vi "SWERVE_TRAJECTORY_BEGIN.vi"(10 "gyroAngle":T2={"VALUE"=0.0, "COS"=1.0, "SIN"=0.0} {"SIN" format="%13.4f"; "COS" format="%13.4f"; "VALUE" format="%13.4f"}, 11 "Module Positions":T1[](array[typedef]) {"Angle"."SIN" format="%13.4f"; "Angle"."COS" format="%13.4f"; "Angle"."VALUE" format="%13.4f"}) -> ()   [LabVIEW 2019]
uses:
  <vilib>/Rock Robotics/WPI/ThirdParty/JAS_Junk/TrajLib/Trajectory_Library.lvlib
  SWERVE_TRAJECTORY_GLOBALS.vi
  <vilib>/Rock Robotics/WPI/ThirdParty/JAS_Junk/TrajLib/TypeDef/ROTATION2D.ctl
  <vilib>/Rock Robotics/WPI/ThirdParty/JAS_Junk/TrajLib/TypeDef/SWERVE_DRIVE_MODULE_POSITION.ctl
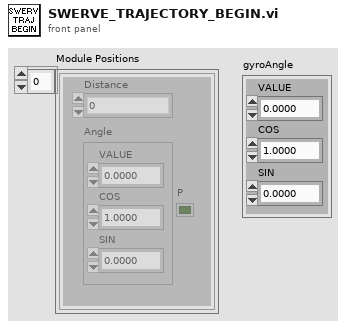
[diagram p1: front panel]
types:
  T1 = typedef "Trajectory_Library.lvlib/SWERVE_DRIVE_MODULE_POSITION.ctl" = cluster{"Distance":dbl, "Angle":T2, "P":bool}
  T2 = typedef "Trajectory_Library.lvlib/ROTATION2D.ctl" = cluster{"VALUE":dbl, "COS":dbl, "SIN":dbl}
  T3 = typedef "Trajectory_Library.lvlib/SWERVE_DRIVE_ODOMETRY.ctl" = cluster{"POSE":T4, "GyroOffset":T2, "PreviousAngle":T2, "PrevModulePositions":T1[], "NumModules":i32}
  T4 = typedef "Trajectory_Library.lvlib/POSE2D.ctl" = cluster{"TRANSLATION":T5, "ROTATION":T2}
  T5 = typedef "Trajectory_Library.lvlib/TRANSLATION2D.ctl" = cluster{"X":dbl, "Y":dbl}
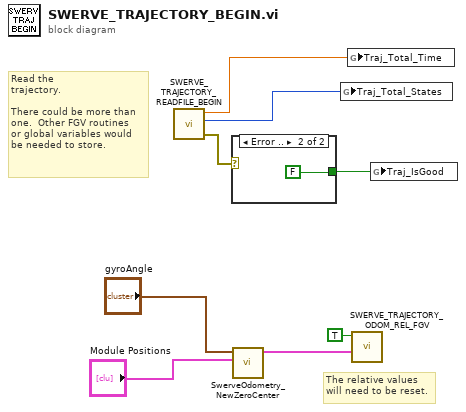
[diagram p0: block diagram]
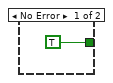
[diagram p2: hidden frame]
diagram:
  # "The relative values\nwill need to be reset."
  # "Read the\ntrajectory.\n\nThere could be more than\none.  Other FGV routines\nor global variables would\nbe needed to store."
  n1 = call "SWERVE_TRAJECTORY_READFILE_BEGIN.vi"() -> ("error out"=w8:errorcluster, "Trajectory Items"=w2:i32, "TotalTImeSecs"=w3:dbl)  [unwired: 9 in]
  n2 = case shown="Error .." w8 {
    tunnel: [TRUE FALSE] -> w1
    frame No Error {
    }
    frame Error {
    }
  }
  n3 = call <vilib>:"SwerveOdometry_NewZeroCenter.vi"("Module Positions"="Module Positions", "gyroAngle"="gyroAngle") -> ("SWERVE_DRIVE_ODOMETRY"=w7:T3)  [unwired: 9 in]
  n4 = global write "SWERVE_TRAJECTORY_GLOBALS.vi" "Traj_Total_States"(w2) -> ()
  n5 = global write "SWERVE_TRAJECTORY_GLOBALS.vi" "Traj_Total_Time"(w3) -> ()
  n6 = call "SWERVE_TRAJECTORY_ODOM_REL_FGV.vi"("in SWERVE_DRIVE_ODOMETRY"=w7, "WRITE"=TRUE) -> ()  [unwired: 9 in, 1 out]
  n7 = global write "SWERVE_TRAJECTORY_GLOBALS.vi" "Traj_IsGood"(w1) -> ()
